vi "octave_cmd_get_version.vi"(5 "recieve interval [ms]":i32=100, 7 "timeout [ms]":i32=1000, 8 "error in":errorcluster, 11 "instance handle in":u32[](array[numeric])) -> (0 "error out":errorcluster, 2 "version string":string, 3 "instance handle out":u32[](array[numeric]))   [LabVIEW 2011]
doc: "Tries to read out GNU Octave version by means of 'ver' command.\nIf no process instance handle is connected, last one from global variable is used or new instance handle is stored to it."
uses:
  <vilib>/regexp/Match Regular Expression.xnode
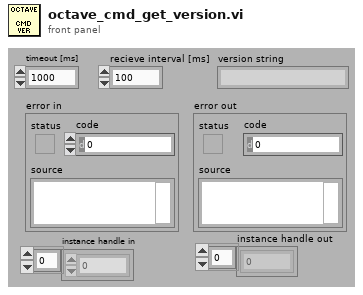
[diagram p1: front panel]
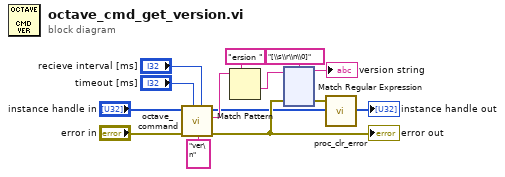
[diagram p0: block diagram]
diagram:
  n1 = call "octave_command.vi"("recieve interval [ms]"="recieve interval [ms]", "timeout [ms]"="timeout [ms]", "error in"="error in", "write buffer"="ver\n", "instance handle in"="instance handle in") -> ("error out"=w7:errorcluster, "read buffer"=w3:string, "instance handle out"=→"instance handle out":u32[])  [unwired: 2 in, 2 out]
  "error out" <- w7
  n2 = Match Pattern(string=w3, regular expression="ersion ") -> (after substring=w10:string)  [unwired: 1 in, 3 out]
  n3 = xnode "Match Regular Expression"("input string"=w10, "regular expression"="[\\s\\r\\n\\0]", "error in"=w7) -> ("before match"=→"version string":string, "error out"=w9:errorcluster)  [unwired: 3 in, 3 out]
  n4 = call "proc_clr_error.vi"("error in (no error)"=w9) -> ()  [unwired: 4 in, 1 out]
